vi "Available Exposure Modes.vi"(8 "error in (no error)":errorcluster, 11 "Camera in":refnum<class "Camera.lvclass">) -> (0 "error out":errorcluster, 2 "Exposure Modes":T1[](array[typedef]), 3 "Camera":refnum<class "Camera.lvclass">)   [LabVIEW 2020, in "Camera.lvclass"]
uses:
  Camera.lvclass
  Exposure Mode.ctl
  Camera.lvclass/Camera.ctl
  1d0181f0-64a9-471c-9d08-be33338c9a07.vi
  84d87f68-00df-4f07-8889-951d30b90fde.vi
  Check Not Disconnected.vi
  <vilib>/Utility/error.llb/Error Cluster From Error Code.vi
  <vilib>/Comparison/Equal/Equal Functor/Equal Functor.lvclass
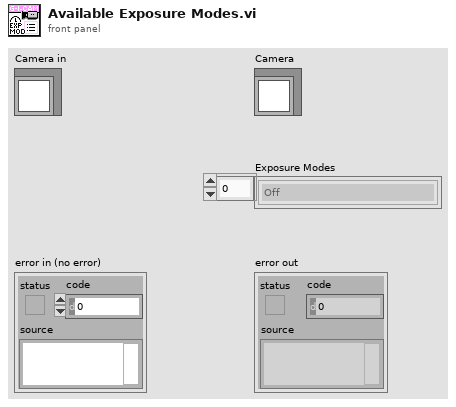
[diagram p1: front panel]
types:
  T1 = typedef "Camera.lvclass/Exposure Mode.ctl" = enum8{"Off", "Timed", "Trigger Width", "Trigger Controller"}
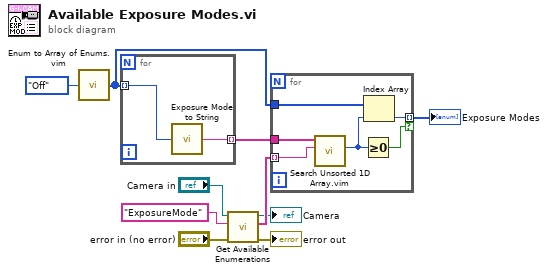
[diagram p0: block diagram]
diagram:
  n1 = call "Enum to Array of Enums.vim"("enum"=Exposure_Mode."Off" ("Exposure Mode")) -> ("array of enums"=w6:T1[])
  n2 = for {
    tunnel: w6 -> [w12] mode=indexing
    tunnel: [w11] -> w7 mode=indexing
    n3 = call "Exposure Mode to String.vi"("Exp Mode"=w12) -> ("String"=w11:string)
  }
  n4 = call "Get Available Enumerations.vi"("error in (no error)"="error in (no error)", "Feature"="ExposureMode" ("Name"), "Camera in"="Camera in") -> ("error out"=→"error out":errorcluster, "Available Enumerations"=w4:string[], "Camera"=→"Camera":refnum<class "Camera.lvclass">)  [unwired: 6 in]
  n5 = for {
    tunnel: w7 -> [w18]
    tunnel: w6 -> [w17]
    tunnel: w4 -> [w16] mode=indexing
    tunnel: [w15] -> w3 mode=indexing if=w13
    n6 = call "Search Unsorted 1D Array.vim"("element"=w16, "unsorted 1D array"=w18) -> ("index of element"=w14:i32)  [unwired: 9 in]
    n7 = Greater Or Equal To 0?(x=w14) -> (x >= 0?=w13:bool)
    n8 = Index Array(array=w17, index=w14) -> (element=w15:T1)
  }
  "Exposure Modes" <- w3
